vi "Generate Expanding Scan Squares.vi"() -> ()   [LabVIEW 2020, in "Bubble.lvclass"]
uses:
  Bubble.lvclass
panel:
  out "Array":cluster{i32[], i32[]}[](array[cluster])
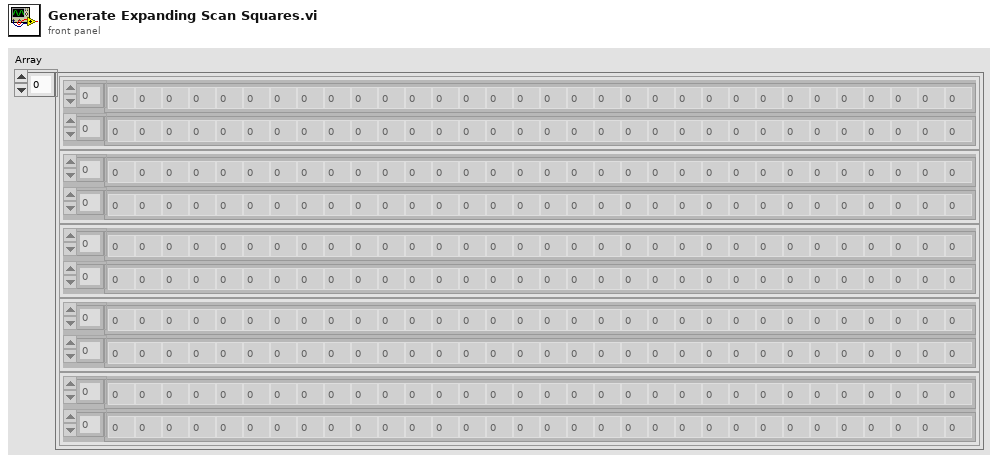
[diagram p1: front panel]
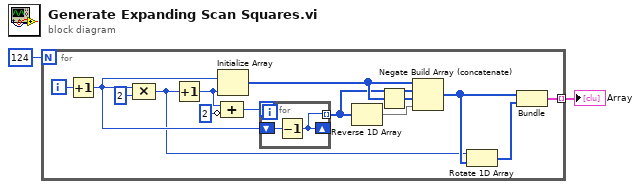
[diagram p0: block diagram]
diagram:
  n1 = for {
    N: 124 -> [_]
    tunnel: [w4] -> w1 mode=indexing
    i -> [w16]
    n2 = Increment(x=w16) -> (x+1=w13:i32)
    n3 = Compound Arithmetic op=MULTIPLY(w13, 2 ("value")) -> (w5:i32)
    n4 = Increment(x=w5) -> (x+1=w14:i32)
    n5 = Initialize Array(w13, w14) -> (w11:i32[])
    n6 = Compound Arithmetic op=ADD(w14, invert 2 ("value")) -> (w9:i32)
    n7 = for {
      N: w9 -> [_]
      shift-right: [w17] -> _
      shift-left: w13 -> [w18]
      tunnel: [w17] -> w3 mode=indexing
      n8 = Decrement(x=w18) -> (x-1=w17:i32)
    }
    n9 = Reverse 1D Array(array=w3) -> (reversed array=w8:i32[])
    n10 = Negate(x=w11) -> (-x=w12:i32[])
    n11 = Build Array (concatenate)(w11, w3, w12, w8) -> (w7:i32[])
    n12 = Rotate 1D Array(1:w7, 2:w5) -> (0:w6:i32[])
    n13 = Bundle(w7, w6) -> (w4:cluster{i32[], i32[]})  [unwired: 1 in]
  }
  "Array" <- w1
